vi "resetBitS0_32.vi"(8 "error in (no error)":errorcluster, 9 "Address":u8, 10 "bitnumber":u32) -> (0 "error out":errorcluster)   [LabVIEW 2015, in "ESLSCDLL.lvlib"]
uses:
  ESLSCDLL.lvlib
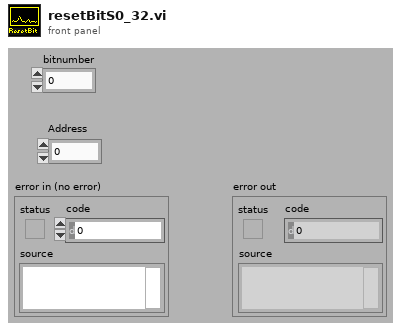
[diagram p1: front panel]
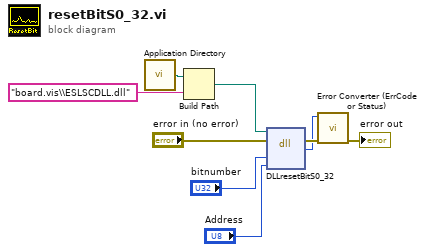
[diagram p0: block diagram]
diagram:
  n1 = call <vilib>:"Application Directory.vi"() -> ("Application Directory"=w3:path)
  n2 = Build Path(base path=w3, name or relative path="board.vis\\ESLSCDLL.dll") -> (appended path=w1:path)
  n3 = dll-call lib="C:/ENTW/PCIE/LV64/board.vis/ESLSCDLL.dll" fn="DLLresetBitS0_32" ("lwlscdll.dll:DLLRsTOREG")(path in=w1, error in="error in (no error)", "bitnumber"="bitnumber", "Address"="Address") -> (error out=w5:errorcluster, "es_status_codes"=w4:i32)  [unwired: 3 in, 1 out]
  n4 = call "Error Converter (ErrCode or Status).vi"("error in (no error)"=w5, "error code"=w4) -> ("error out"=→"error out":errorcluster)  [unwired: 9 in]
